vi "WaitForConnection.vi"(8 "error in (no error)":errorcluster, 11 "Tcp in":refnum<class "Tcp.lvclass">) -> (0 "error out":errorcluster, 3 "Tcp out":refnum<class "Tcp.lvclass">)   [LabVIEW 2022 SP3, in "Tcp.lvlib" / "Tcp.lvclass"]
uses:
  Tcp.lvclass
  C:/Program Files (x86)/National Instruments/LabVIEW 2022/vi.lib/ActorFramework/Actor/Actor.lvclass
  Tcp.lvclass/Tcp.ctl
  Connection/Connection/Connection.lvclass
  TcpSocket/Source/TcpSocket/Connection/Connection.lvclass/Connection.ctl
  Connection/Connection Messages/Initialize Msg/Initialize Msg.lvclass/Initialize Msg.ctl
  <vilib>/ActorFramework/Message Enqueuer/Message Enqueuer.lvclass/Message Enqueuer.ctl
  <vilib>/ActorFramework/Actor/Actor.lvclass/Actor.ctl
  TcpSocket/Source/TcpSocket/Connection/Read Connection.vi
  <vilib>/ActorFramework/Message Enqueuer/Enqueue.vi
  <vilib>/ActorFramework/Message Enqueuer/Init from Existing Queue.vi
  Connection/Connection Messages/Initialize Msg/Initialize Msg.lvclass
  C:/Program Files (x86)/National Instruments/LabVIEW 2022/vi.lib/ActorFramework/Message/Message.lvclass
  Tcp Messages/WaitForConnection Msg/WaitForConnection Msg.lvclass
  <vilib>/ActorFramework/Message Priority Queue/Priority Enqueue.vi
  <vilib>/ActorFramework/Message Enqueuer/Message Enqueuer.lvclass
  TcpSocket/Source/TcpSocket/TcpServer/TcpServer.lvclass
  Logger/Source/Logger/Logger.lvclass
  <vilib>/ActorFramework/Actor/Actor.lvclass
  C:/Users/jakub/repos/gh/sw4sys/lv-cli-framework/LoggingActor/Source/LoggingActor/LoggingActor/LoggingActor.lvclass
  C:/Users/jakub/repos/gh/sw4sys/lv-cli-framework/CliFramework/Source/Tcp/Tcp/Tcp.lvclass
  C:/Users/jakub/repos/gh/sw4sys/lv-cli-framework/CliFramework/Source/Connection/CallerMessage/CallerMessage.lvclass
  TcpSocket/Source/TcpSocket/Connection/Connection.lvclass
  C:/Users/jakub/repos/gh/sw4sys/lv-cli-framework/CliFramework/Source/Connection/Connection/Connection.lvclass
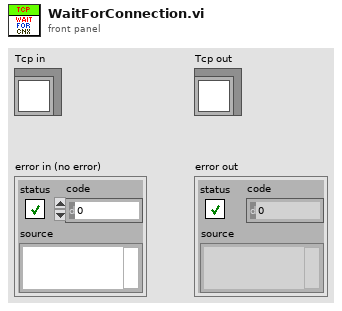
[diagram p1: front panel]
types:
  T1 = map{u64, refnum<class "Message Enqueuer.lvclass">}
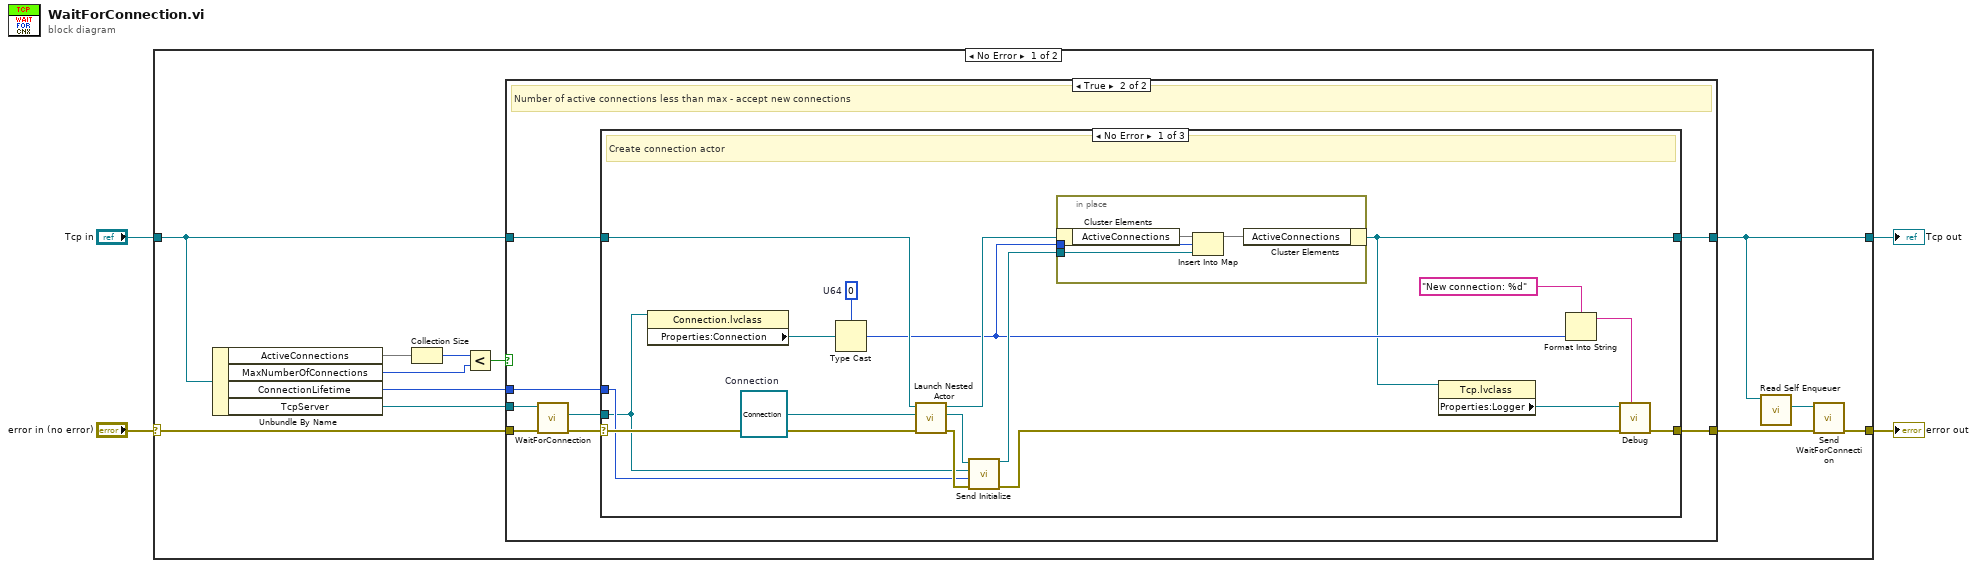
[diagram p0: block diagram]
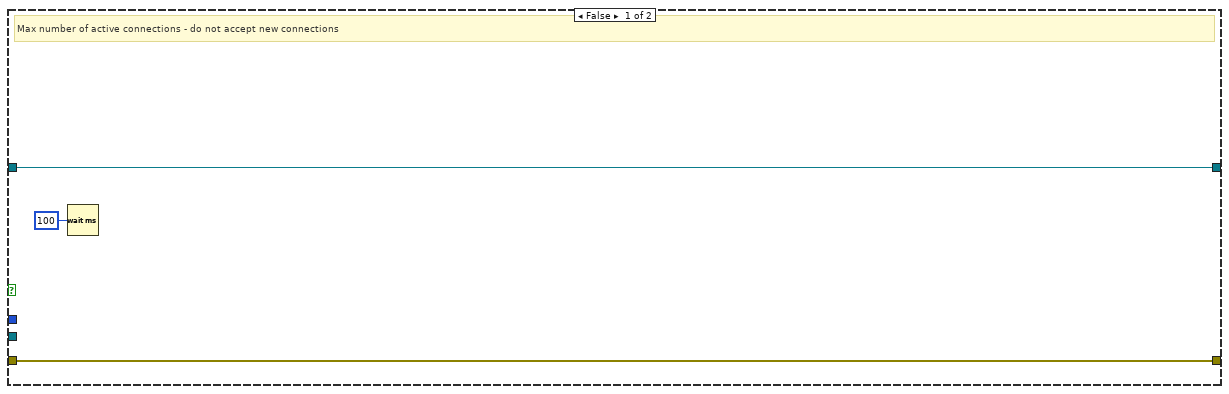
[diagram p2: hidden frame]
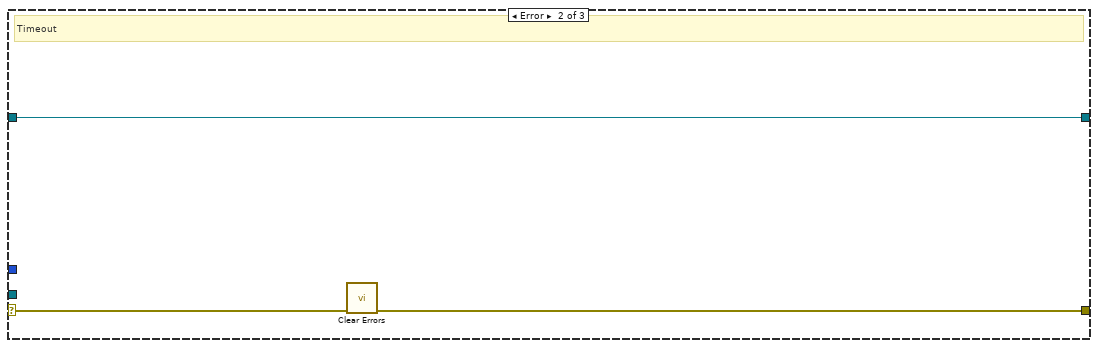
[diagram p3: hidden frame]
diagram:
  n1 = case shown="No Error" "error in (no error)" {
    selector: "error in (no error)" -> [w16 w56]
    tunnel: [w10 w56] -> w3
    tunnel: [w12 w55] -> w1
    tunnel: "Tcp in" -> [w14 w55]
    frame No Error {
      n2 = Unbundle By Name(w14) -> ("ActiveConnections"=w8:T1, "MaxNumberOfConnections"=w6:i32, "ConnectionLifetime"=w13:i32, "TcpServer"=w15:refnum<class "TcpServer.lvclass">)
      n3 = Collection Size(1:w8) -> (0:w7:i32)
      n4 = Less?(x=w7, y=w6) -> (x < y?=w5:bool)
      n5 = case shown="True" w5 {
        tunnel: w16 -> [w19 w27]
        tunnel: w15 -> [_ w24]
        tunnel: w14 -> [w18 w23]
        tunnel: w13 -> [_ w22]
        tunnel: [w18 w21] -> w12
        tunnel: [w19 w20] -> w11
        frame False {
          # "Max number of active connections - do not accept new connections"
          n6 = Wait (ms)(milliseconds to wait=u32 100) -> ()  [unwired: 1 out]
        }
        frame True {
          # "Number of active connections less than max - accept new connections"
          n7 = call-dynamic "WaitForConnection.vi"("error in (no error)"=w27, "TcpServer in"=w24) -> ("error out"=w26:errorcluster, "Connection"=w25:refnum<class "Connection.lvclass">)  [unwired: 7 in, 1 out]
          n8 = case shown="No Error" w26 {
            selector: w26 -> [w45 w52 w54]
            tunnel: [w33 w50 w54] -> w20
            tunnel: w25 -> [w37 _ _]
            tunnel: w23 -> [w43 w51 w53]
            tunnel: [w29 w51 w53] -> w21
            tunnel: w22 -> [w40 _ _]
            frame No Error {
              w35 = u64 0  # U64
              w44 = refnum<class "Connection.lvclass"> refnum  # Connection
              # "Create connection actor"
              n9 = property class="Connection.lvclass"(reference=w37) -> ("Properties:Connection"=w36:refnum<k5>)  [unwired: 1 in, 2 out]
              n10 = Type Cast(type=w35, x=w36) -> (*(type *) &x=w31:u64)
              n11 = call <vilib>:"Launch Nested Actor.vi"("error in (no error)"=w45, "Nested Actor"=w44, "Caller Actor in"=w43) -> ("error out"=w41:errorcluster, "Nested Actor's Enqueuer"=w42:refnum<class "Message Enqueuer.lvclass">, "Caller Actor out"=w38:refnum<class "Tcp.lvclass">)  [unwired: 6 in]
              n12 = call "Send Initialize.vi"("error in (no error)"=w41, "Timeout [ms] (5000)"=w40, "Connection"=w37, "Message Enqueuer"=w42) -> ("error out"=w34:errorcluster, "Message Enqueuer out"=w39:refnum<class "Message Enqueuer.lvclass">)  [unwired: 6 in]
              n13 = in-place {
                in-place-border: w39 -> [w47]
                in-place-border: w31 -> [w46]
                n14 = in-place-cluster #1(w38) -> ("ActiveConnections"=w49:T1)
                n15 = Insert Into Map(map in=w49, key=w46, value=w47) -> (map out=w48:T1)  [unwired: 2 out]
                n16 = in-place-cluster #1("ActiveConnections"=w48) -> (w29:refnum<class "Tcp.lvclass">)
              }
              n17 = property class="Tcp.lvclass"(reference=w29) -> ("Properties:Logger"=w28:refnum<class "Logger.lvclass">)  [unwired: 1 in, 2 out]
              n18 = Format Into String(format string="New connection: %d", w31) -> (resulting string=w30:string)  [unwired: 2 in, 1 out]
              n19 = call-dynamic "Debug.vi"("Message"=w30, "error in (no error)"=w34, "Logger in"=w28) -> ("error out"=w33:errorcluster)  [unwired: 7 in, 1 out]
            }
            frame Error {
              # "Timeout"
              n20 = call <vilib>:"Clear Errors.vi"("error in (no error)"=w52) -> ("error out"=w50:errorcluster)  [unwired: 5 in, 1 out]
            }
            frame Default {
              # "Error"
            }
          }
        }
      }
      n21 = call <vilib>:"Read Self Enqueuer.vi"("Actor"=w12) -> ("Self Enqueuer"=w9:refnum<class "Message Enqueuer.lvclass">)  [unwired: 10 in]
      n22 = call "Send WaitForConnection.vi"("error in (no error)"=w11, "Message Enqueuer"=w9) -> ("error out"=w10:errorcluster)  [unwired: 8 in, 1 out]
    }
    frame Error {
    }
  }
  "error out" <- w3
  "Tcp out" <- w1
